vi "Set State.vi"(7 "VI Ref":refnum<vi>, 8 "Error":errorcluster, 9 "State":T1(ring)=enum."Standard", 11 "FP":refnum<class "DecFrame_FP.lvclass">) -> (0 "Error Out":errorcluster, 3 "FP Out":refnum<class "DecFrame_FP.lvclass">, 5 "VI Ref":refnum<vi>)   [LabVIEW 2020, in "DecFrame_FP.lvclass"]
uses:
  DecFrame_FP.lvclass
  C:/Users/mark.balla/Documents/~Projects/MB Tools/LabVIEW 2020/Project Template/Utility/Universal Utility/FP/FPClass/FP/FP.lvclass
  TypeDefs_Utility/ENUM RB_Pos_Quadrant Position.ctl
  FP/FP.lvclass
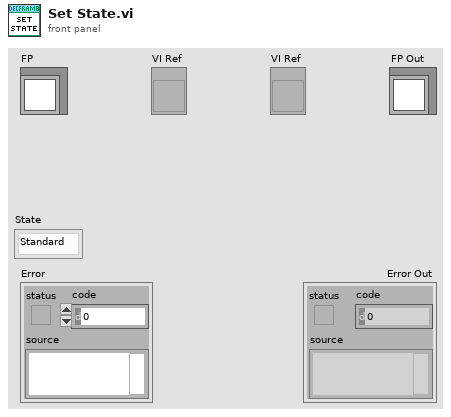
[diagram p1: front panel]
types:
  T1 = enum32{"Invalid", "Standard", "Closed", "Hidden", "Minimized", "Maximized"}
  T2 = typedef "ENUM RB_Pos_Quadrant Position.ctl" = enum32{"LFT-TOP", "MID-TOP", "RGT-TOP", "LFT-CTR", "MID-CTR", "RGT-CTR", "LFT-BOT", "MID-BOT", "RGT-BOT"}
  T3 = enum32{"invalid app kind", "Development System", "Run Time System", "Student Edition", "Embedded LabVIEW", "Evaluation", "Custom"}
  T4 = typedef "LVRectTypeDef.ctl" = cluster{"Left":i16, "Top":i16, "Right":i16, "Bottom":i16}
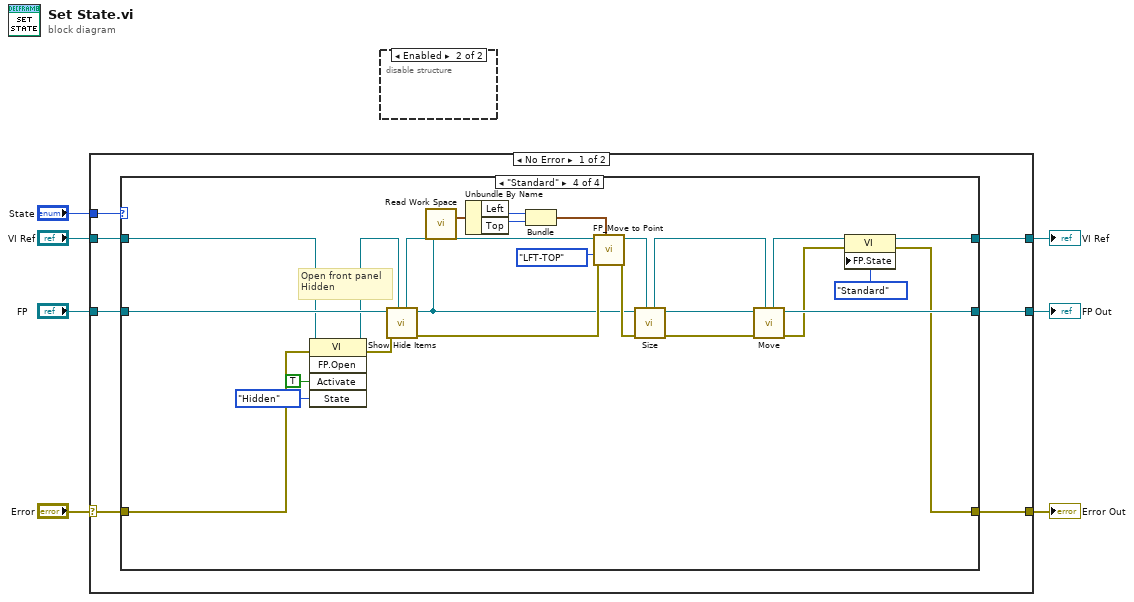
[diagram p0: block diagram]
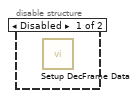
[diagram p2: hidden frame]
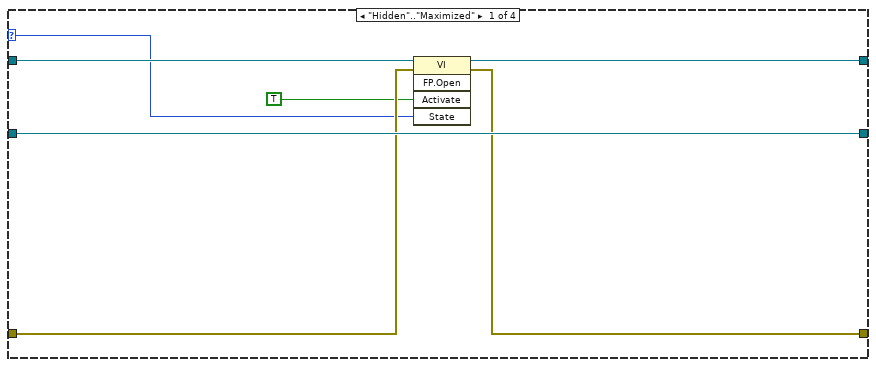
[diagram p3: hidden frame]
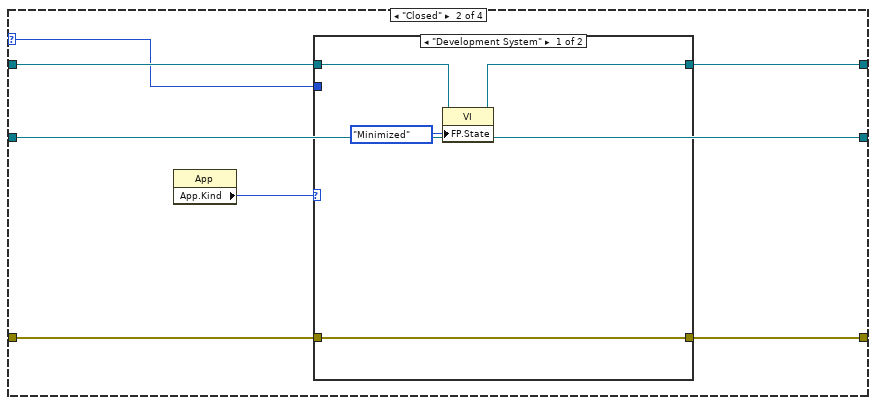
[diagram p4: hidden frame]
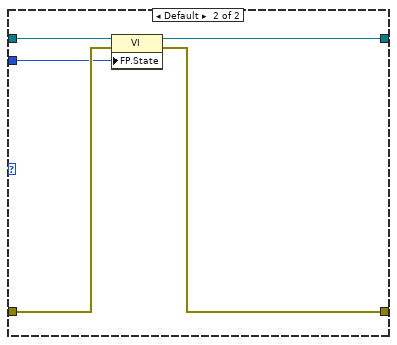
[diagram p5: hidden frame]
diagram:
  n1 = case shown="No Error" "Error" {
    selector: "Error" -> [w11 w69]
    tunnel: [w8 w69] -> w6
    tunnel: [w9 w68] -> w4
    tunnel: "FP" -> [w12 w68]
    tunnel: "VI Ref" -> [w13 w67]
    tunnel: [w10 w67] -> w2
    tunnel: "State" -> [w14 _]
    frame No Error {
      n2 = case shown="\"Standard\"" w14 {
        selector: w14 -> [w15 w23 _ _]
        tunnel: w13 -> [w20 w27 w39 w46]
        tunnel: w12 -> [w21 w28 w40 w62]
        tunnel: w11 -> [w18 w25 w38 w58]
        tunnel: [w19 w26 w39 w48] -> w10
        tunnel: [w21 w28 w40 w54] -> w9
        tunnel: [w17 w24 w38 w50] -> w8
        frame "Hidden".."Maximized" {
          n3 = invoke class="VI" method="FP.Open"(reference=w20, error in=w18, "Activate"=TRUE ("Activate?"), "State"=w15) -> (reference out=w19:refnum<vi>, error out=w17:errorcluster)  [unwired: 1 in, 3 out]
        }
        frame "Closed" {
          n4 = property class="App"() -> ("App.Kind"=w22:T3)  [unwired: 2 in, 2 out]
          n5 = case shown="\"Development System\"" w22 {
            tunnel: w27 -> [w31 w37]
            tunnel: [w30 w36] -> w26
            tunnel: w25 -> [w32 w35]
            tunnel: [w32 w34] -> w24
            tunnel: w23 -> [_ w33]
            frame "Development System" {
              n6 = property class="VI"(reference=w31, "FP.State"=T1."Minimized" ("Front Panel Window:State")) -> (reference out=w30:refnum<vi>)  [unwired: 1 in, 1 out]
            }
            frame Default {
              n7 = property class="VI"(reference=w37, error in=w35, "FP.State"=w33) -> (reference out=w36:refnum<vi>, error out=w34:errorcluster)
            }
          }
        }
        frame "Invalid" {
        }
        frame "Standard" {
          # "Open front panel\nHidden"
          n8 = invoke class="VI" method="FP.Open"(reference=w46, error in=w58, "Activate"=TRUE ("Activate?"), "State"=T1."Hidden") -> (reference out=w59:refnum<vi>, error out=w57:errorcluster)  [unwired: 1 in, 3 out]
          n9 = call-dynamic "Show Hide Items.vi"("VI Ref"=w59, "Error"=w57, "FP"=w62) -> ("Error Out"=w47:errorcluster, "FP Out"=w45:refnum<class "DecFrame_FP.lvclass">, "VI Ref Out"=w66:refnum<vi>)  [unwired: 6 in]
          n10 = call "Read Work Space.vi"("FP"=w45) -> ("WkSpace Out"=w44:T4)  [unwired: 2 in]
          n11 = Unbundle By Name(w44) -> ("Left"=w43:i16, "Top"=w42:i16)
          n12 = Bundle("Left"=w43, "Top"=w42) -> (w41:cluster{"Left":i16, "Top":i16})  [unwired: 1 in]
          n13 = call "FP_Move to Point.vi"("Target Point"=w41, "Error"=w47, "FP Position"=ENUM_RB_Pos_Quadrant_Position."LFT-TOP", "VI"=w66) -> ("Error Out"=w63:errorcluster, "VI Out"=w65:refnum<vi>)  [unwired: 6 in]
          n14 = call "Size.vi"("VI Ref"=w65, "Error"=w63, "DecFrame_FP"=w45) -> ("Error Out"=w53:errorcluster, "DecFrame_FP Out"=w55:refnum<class "DecFrame_FP.lvclass">, "VI Out"=w52:refnum<vi>)  [unwired: 6 in]
          n15 = call "Move.vi"("VI Ref"=w52, "Error"=w53, "DecFrame_FP"=w55) -> ("Error Out"=w51:errorcluster, "DecFrame_FP Out"=w54:refnum<class "DecFrame_FP.lvclass">, "VI Out"=w49:refnum<vi>)  [unwired: 6 in]
          n16 = property class="VI"(reference=w49, error in=w51, "FP.State"=T1."Standard" ("Front Panel Window:State")) -> (reference out=w48:refnum<vi>, error out=w50:errorcluster)
        }
      }
    }
    frame Error {
    }
  }
  "Error Out" <- w6
  "FP Out" <- w4
  "VI Ref" <- w2
  n17 = disable-structure shown="Enabled" {
    frame Disabled {
      n18 = call-dynamic "Setup DecFrame Data.vi"() -> ()  [unwired: 10 in, 2 out]
    }
    frame Enabled {
    }
  }
